vi "T90 main.vi"() -> ()   [LabVIEW 2020, in "T90.lvlib"]
uses:
  T90.lvlib
  Visualisierungs Elemente/Auswahlfeld.ctl
  Visualisierungs Elemente/Zahlen-Ausgabefeld.ctl
  Visualisierungs Elemente/Button.ctl
  Seiten/FT-IR/FGV FT-IR Gasliste Aktionen.ctl
  Aktion FGV T90.ctl
  Seiten/Gaszuordnung AO/FGV Gaszuordnung Grenzen&Einheit Aktion.ctl
  Aktion Zustandsautomat.ctl
  Messdaten/Aktionen FGV Messdaten.ctl
  Schedule Modul/Aktion FGV Testdaten sammeln.ctl
  Funktionstasten/Funktionstasten-Aktion.ctl
  Funktionstasten/Zustaende.ctl
  Funktionstasten/FGV Erweiterte Bedienung Aktion.ctl
  T90 konfig.vi
  Messdaten/Messdaten.lvlib
  Seiten/FT-IR/FT-IR.lvlib
  Allgemein/allgemeine Sub-VIs.lvlib
  Funktionstasten/Funktionstasten.lvlib
  Seiten/Gaszuordnung AO/Gaszuordnung AO.lvlib
  Sprachverwaltung/Sprachverwaltung.lvlib
  Linearisierung V2/Protokoll/Protokoll.lvlib
  Schedule Modul/Schedule Modul.lvlib
  cRIO/PC/Kommunikation mit cRIO.lvlib
panel:
  out "T90 PDF":waveform(sgl)(graph) caption="T90"
  out "Einheit 2":string caption="Einheit"
  out "Durchfluss FTIR":T1 format="%#.3g"
  out "Bestanden?":bool caption="Ergebnis 1"
  out "Ergebnis:":string
  out "T50:":T1 caption="T50 (Response Time):" format="%#.2g"
  out "Rise Time":T1 caption="T10 - T90 (Rise Time):" format="%#.1g"
  out "T90:":T1 caption="T90 (Response Time):" format="%#.1g"
  out "T10:":T1 caption="T10 (Delay Time):" format="%#.2g"
  out "Status":string
  out "Einheit":string
  out "aktuelle Wert":T1 caption="aktueller Wert" format="%#.3g"
  in  "Abbrechen":T2
  out "Gaskomponente":T3 caption="Komponente" items=["NO (350,3000) LP 191C", "NO2 (150) LP 191C (1of2)", "NO2 (2000) LP 191C (2of2)", "N2O (300) LP 191C (1of2)", "NH3 (300) LP 191C (1of2)", "NH3 (900,3000) LP 191C (2of2)", "HNCO (400) 191C", "H2O% (30) LP 191C", "Formaldehyde (70,500) LP 191C", "CO2 low% (4) LP 191C (2of2)", "CO2% (20) LP 191C (1of2)", "CO (700) LP 191C (1of3)", "CO% (1) LP 191C (2of3)", "Propylene (1000) LP 191C", "Aromatic HC C7 (500) LP 191C", "Ethylene (1000) LP 191C", "CH4 (250) LP 191C (1of2)", "CH4 (5000) LP 191C (2of2)", "Ethane (1000) LP 191C", "Acetylene (1000) LP 191C", "HNO2 (20) 191C", "MeOH (1000) 191C", "CO% (10) LP 191C (3of3)", "Formic Acid (100) 191C", "SO2 (500) LP 191C", "Acetaldehyde (1000) LP 191C", "COS (100) LP 191C", "1,3 butadiene (100) LP 191C", "Oil as Octane (200) LP 191C", "N2O (1000) LP 191C (2of2)", "Propane (200) LP 191C", "NO2 autorange (2000)", "CO autorange (100000)", "CH4 autorange (5000)", "NH3 autorange (3000)", "NOx autorange (3000)", "HCD (10000)", "NMHCD (10000)", "CO2% autorange (20)", "H2Oppm (300000)", "N2O autorange (1000)", "NMNEHCD (3000)", "Temp. Messzelle", "Druck Messzelle", "sBeam@2500", "Temp. HL zu FT-IR", "Temp. HL Extern SP1", "Austrittstemp. FT-IR", "Temp. Schaltschrank", "Konstant 0", "Konstant 50", "Konstant 100", "AK DUMMY"]
  out "T90":waveform(sgl)(graph)
  # "sec."
  # "sec."
  # "sec."
  # "sec."
  # "T90"
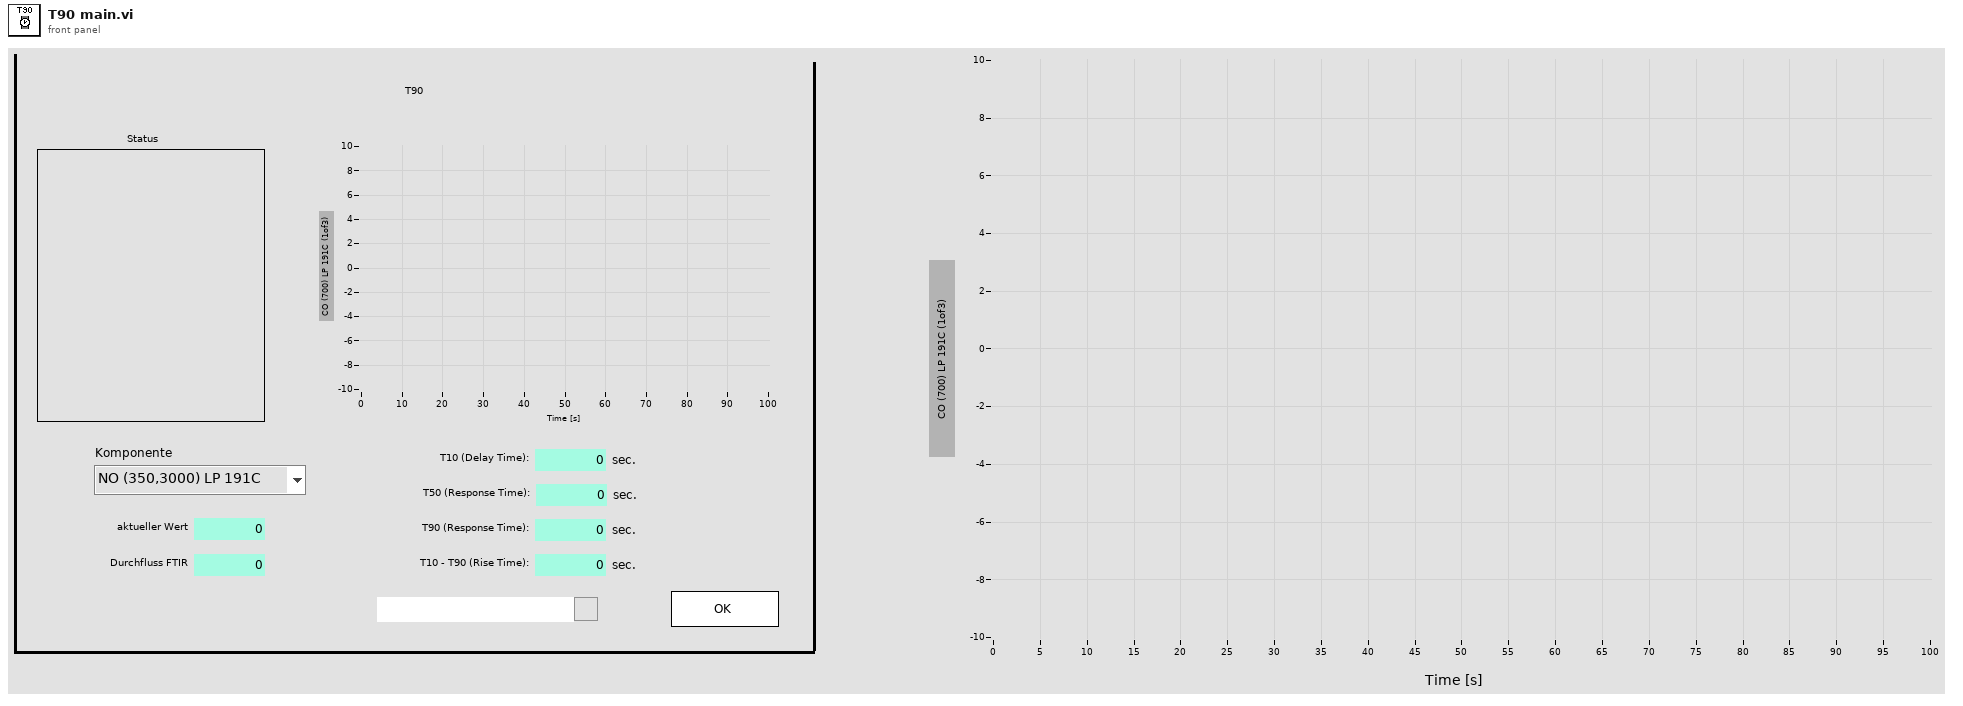
[diagram p1: front panel]
types:
  T1 = typedef "Zahlen-Ausgabefeld.ctl" = sgl
  T2 = typedef "Button.ctl" = bool
  T3 = typedef "Auswahlfeld.ctl" = u16
  T4 = typedef "Gaszuordnung AO.lvlib/FGV Gaszuordnung Grenzen&Einheit Aktion.ctl" = enum16{"Lesen", "Schreiben Min", "Schreiben Max", "Laden", "Speichern"}
  T5 = typedef "T90.lvlib/Aktion FGV T90.ctl" = enum16{"lesen", "schreiben", "laden", "speichern", "T90 aktiv", "T90 Entnahme aktiv", "Overflow Leak", "Pfad", "Zustand", "max. Responsetime"}
  T6 = typedef "FT-IR.lvlib/FGV FT-IR Gasliste Aktionen.ctl" = enum16{"lesen", "Gasliste FT-IR", "Gasliste ausgelesen", "laden", "speichern", "löschen"}
  T7 = typedef "T90.lvlib/Aktion Zustandsautomat.ctl" = enum16{"Initialisieren", "Warten", "Gas aufschalten", "Stabilisieren", "Volle Konzentration 1", "Berechnen", "Prüfung starten", "Prüfung", "Prüfung beenden", "keine Funktion"}
  T8 = typedef "T90.lvlib/T90 Gas Konfig.ctl" = cluster{"Gasflasche":T9, "Konfig Gasflasche":T10, "Auswahl":T3, "Sollwert":T11, "Abweichung":T11, "max. Responsetime":T11, "Modus:":T12, "Abschaltzeit":T11, "Stabilisierungszeit":T11, "Bearbeiter":string}
  T9 = typedef "System Einstellungen V2.lvlib/Gasflasche Auswahl.ctl" = u16
  T10 = typedef "System Einstellungen V2.lvlib/Konfig Gasflasche.ctl" = bool
  T11 = typedef "Zahlen-Eingabefeld.ctl" = sgl
  T12 = typedef "T90.lvlib/Zustand Auswahl.ctl" = u16
  T13 = typedef "String - Ausgabefeld.ctl" = string
  T14 = typedef "Messdaten.lvlib/Aktionen FGV Messdaten.ctl" = enum16{"lesen", "schreiben", "löschen", "Mittelwerte", "Komponente"}
  T15 = typedef "Schedule Modul.lvlib/Aktion FGV Testdaten sammeln.ctl" = enum16{"lesen", "Dichtheitstest", "CalGasTest", "T90", "Kalibrieren", "init", "Kalender Daten"}
  T16 = typedef "Verwaltung - cRIO.lvlib/Analog Eingaenge.ctl" = cluster{"AI0: Durchfluss FT-IR":sgl, "AI1: Druck Ausgang":sgl, "AI2: Umgebungsdruck":sgl, "AI3: Druck FT-IR":sgl, "AI4: Druck CalGas":sgl, "AI5: Reserve":sgl, "AI6: Reserve":sgl, "AI7: Reserve":sgl, "Rohwert Durchfluss FT-IR":sgl, "Rohwert Druck Ausgang":sgl, "Rohwert Umgebungsdruck":sgl, "Rohwert Druck FT-IR":sgl, "Rohwert Druck CalGas":sgl, "Rohwert AI5":sgl, "Rohwert AI6":sgl, "Rohwert AI7":sgl, "Rohwert Diffdruck mbar FTIR":sgl}
  T17 = cluster{"Signalverlauf":waveform(sgl), "T90":dbl, "T50":dbl, "T10":dbl, "Rise time ":dbl, "Bestanden?":bool}
  T18 = typedef "Schedule Modul.lvlib/Ergebnis T90.ctl" = cluster{"T90":waveform(sgl), "T10:":T1, "T50:":T1, "T90:":T1, "Rise Time":T1, "Leitungslänge":T11, "Fehler":bool}
  T19 = typedef "Funktionstasten.lvlib/FGV Erweiterte Bedienung Aktion.ctl" = enum16{"Lesen", "Initialisieren", "N2 zu PNS", "Chart wechsel"}
  T20 = typedef "Funktionstasten.lvlib/Zustaende.ctl" = enum16{"Standby", "Pause", "Eco", "Messen", "Kalibrieren", "Spülen Filter", "Spülen Leitung", "Umgebungsluft", "0-Gas", "Cal-Gas", "CG zu PNS", "-------------", "Init 1", "Init 2", "Init 3", "Init 4", "Messen vorbereiten", "Messen durchführen", "Exit"}
  T21 = typedef "Funktionstasten.lvlib/Funktionstasten-Aktion.ctl" = enum16{"Initialisieren", "Zustand setzen", "Taste gedrückt", "Fehler speichern", "Lesen", "Manuell", "Remote", "Bitparallel", "Samplepoint", "Zeit Prüfen", "reset Umschalten"}
  T22 = typedef "String - Eingabefeld.ctl" = string
  T23 = typedef "Pfad-Eingabefeld.ctl" = path
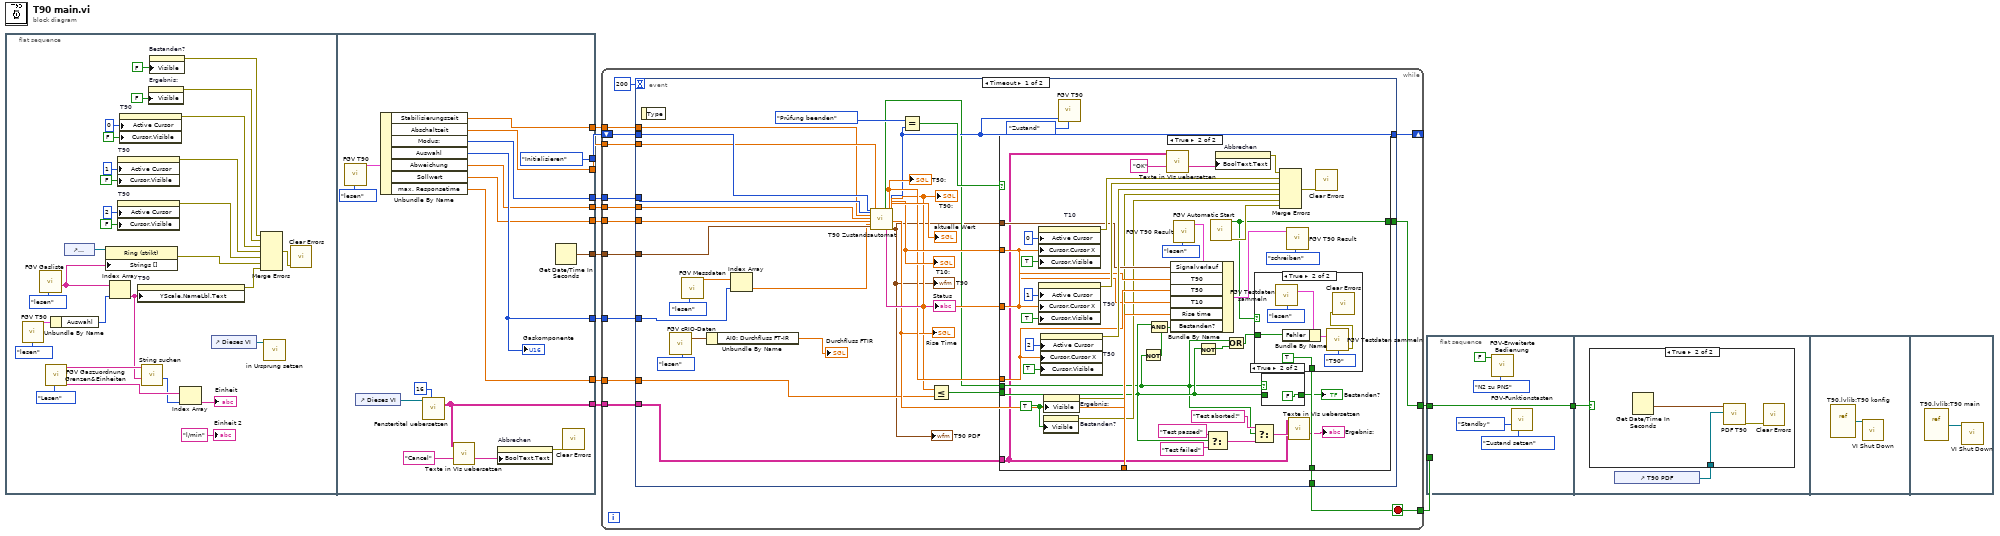
[diagram p0: block diagram]
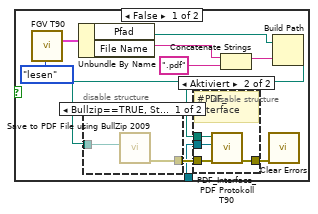
[diagram p2: hidden frame]
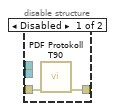
[diagram p3: hidden frame]
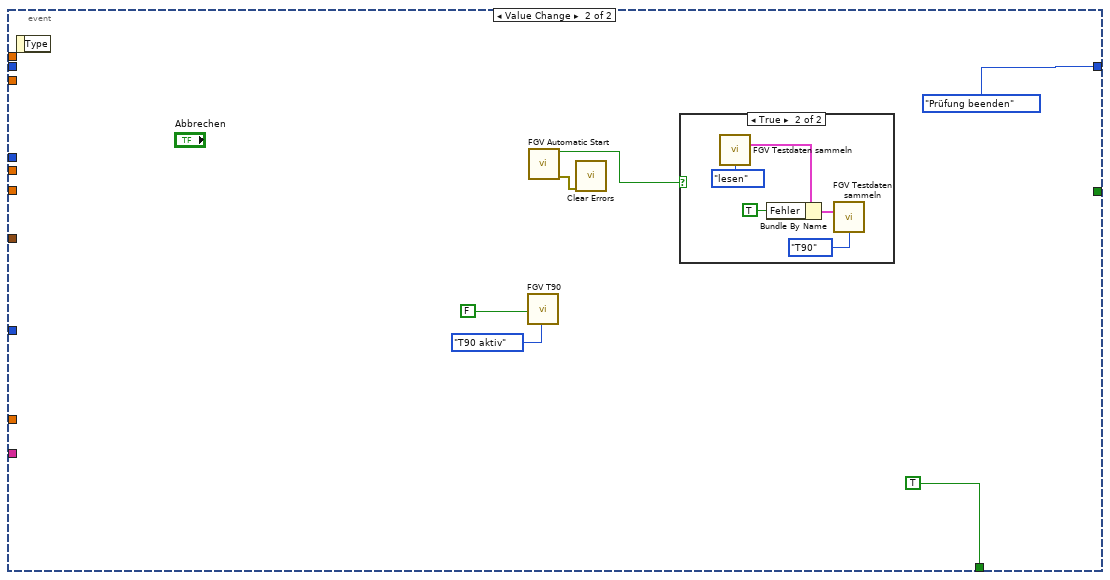
[diagram p8: hidden frame]
diagram:
  n1 = flat-sequence {
    tunnel: [w53] -> w13
    tunnel: [w51] -> w12
    tunnel: [w50] -> w11
    tunnel: [w59] -> w10
    tunnel: [w52] -> w9
    tunnel: [Aktion_Zustandsautomat."Initialisieren" ("Zustand")] -> w7
    tunnel: [w54] -> w6
    tunnel: [w49] -> w5
    tunnel: [w47] -> w4
    tunnel: [w44] -> w1
    frame #0 {
      n2 = call "FGV T90.vi"("Aktion"=Aktion_FGV_T90."lesen") -> ("Gas Konfig"=w16:T8)  [unwired: 20 in, 6 out]
      n3 = call "FGV Gasliste.vi"("Aktionen"=FGV_FT-IR_Gasliste_Aktionen."lesen") -> ("Aktuelle Gasliste gesamt"=w40:T13[])  [unwired: 8 in, 2 out]
      n4 = call "FGV Gaszuordnung Grenzen&Einheiten.vi"("Aktion"=FGV_Gaszuordnung_Grenzen&Einheit_Aktion."Lesen") -> ("Einheit neu"=w30:string[], "Namen neu"=w23:string[])  [unwired: 7 in, 2 out]
      n5 = Unbundle By Name(w16) -> ("Auswahl"=w15:T3)
      n6 = control-ref of="Gaskomponente"() -> (w42:refnum<vi>)
      n7 = property class="Ring (strikt)"(reference=w42, "Strings []"=w40) -> (error out=w38:errorcluster)  [unwired: 1 in, 1 out]
      n8 = Index Array(array=w40, index=w15) -> (element=w22:T13)
      n9 = property on="T90" class="SVGraph (strikt)"("Active Cursor"=u32 1 ("Aktiver Cursor"), "Cursor.Visible"=FALSE ("Cursor.Sichtbar")) -> (error out=w25:errorcluster)  [unwired: 2 in, 1 out]
      n10 = property on="T90" class="SVGraph (strikt)"("Active Cursor"=u32 2 ("Aktiver Cursor"), "Cursor.Visible"=FALSE ("Cursor.Sichtbar")) -> (error out=w26:errorcluster)  [unwired: 2 in, 1 out]
      n11 = property on="T90" class="SVGraph (strikt)"("Active Cursor"=u32 0 ("Aktiver Cursor"), "Cursor.Visible"=FALSE ("Cursor.Sichtbar")) -> (error out=w24:errorcluster)  [unwired: 2 in, 1 out]
      n12 = property on="T90" class="SVGraph (strikt)"("YScale.NameLbl.Text"=w22) -> (error out=w39:errorcluster)  [unwired: 2 in, 1 out]
      n13 = call "String suchen.vi"("Gasname"=w22, "Such-Namen"=w23) -> ("Index"=w21:i32)  [unwired: 8 in, 1 out]
      n14 = property on="Ergebnis:" class="Str"("Visible"=FALSE ("Sichtbar")) -> (error out=w20:errorcluster)  [unwired: 2 in, 1 out]
      n15 = property on="Bestanden?" class="Bool. (strikt)"("Visible"=FALSE ("Sichtbar")) -> (error out=w19:errorcluster)  [unwired: 2 in, 1 out]
      n16 = Index Array(array=w30, index=w21) -> (element=→"Einheit":string)
      n17 = control-ref of="Dieses VI"() -> (w32:refnum<vi>)
      n18 = Merge Errors(w19, w20, w24, w25, w26, w38, w39) -> (w37:errorcluster)
      n19 = call "in Ursprung setzen.vi"("VI Referenz"=w32) -> ()  [unwired: 10 in, 1 out]
      n20 = call <vilib>:"Clear Errors.vi"("error in (no error)"=w37) -> ()  [unwired: 5 in, 2 out]
      "Einheit 2" <- "l/min" ("Einheit 2")
    }
    frame #1 {
      n21 = call "FGV T90.vi"("Aktion"=Aktion_FGV_T90."lesen") -> ("Gas Konfig"=w55:T8)  [unwired: 20 in, 6 out]
      n22 = control-ref of="Dieses VI"() -> (w57:refnum<vi>)
      n23 = Unbundle By Name(w55) -> ("Stabilisierungszeit"=w44:T11, "Abschaltzeit"=w54:T11, "Modus:"=w53:T12, "Auswahl"=w52:T3, "Abweichung"=w51:T11, "Sollwert"=w50:T11, "max. Responsetime"=w49:T11)
      "Gaskomponente" <- w52
      n24 = call "Fenstertitel uebersetzen.vi"("Index (Seite)"=16, "Dieses VI"=w57) -> ("Sprachliste"=w47:string[][])  [unwired: 6 in, 3 out]
      n25 = call "Texte in VIs uebersetzen.vi"("Sprachliste"=w47, "String zum Übersetzen"="Cancel" ("Boolescher Text.Text")) -> ("String zum Übersetzen"=w45:string)  [unwired: 9 in, 4 out]
      n26 = property on="Abbrechen" class="Bool."("BoolText.Text"=w45) -> (error out=w46:errorcluster)  [unwired: 2 in, 1 out]
      n27 = Get Date/Time In Seconds() -> (seconds since 1Jan1904=w59:timestamp)
      n28 = call <vilib>:"Clear Errors.vi"("error in (no error)"=w46) -> ()  [unwired: 5 in, 2 out]
    }
  }
  n29 = while {
    shift-right: [w73] -> _
    shift-left: w7 -> [w72]
    tunnel: w13 -> [w71]
    tunnel: w12 -> [w70]
    tunnel: w11 -> [w69]
    tunnel: w10 -> [w68]
    tunnel: w9 -> [w67]
    tunnel: [w66] -> w8
    tunnel: w6 -> [w65]
    tunnel: w5 -> [w64]
    tunnel: w4 -> [w63]
    tunnel: [w62] -> w3
    tunnel: w1 -> [w61]
    stop <- w66 stop-if-true
    n30 = event shown="[0] Timeout" {
      selector: _ -> [_ _]
      dyn-events: _ -> [_ _]
      timeout: 200 -> [_ _]
      tunnel: [w85 TRUE] -> w66
      tunnel: [w82 Aktion_Zustandsautomat."Prüfung beenden" ("Zustand")] -> w73
      tunnel: w72 -> [w105 _]
      tunnel: w71 -> [w80 _]
      tunnel: w70 -> [w103 _]
      tunnel: w69 -> [w102 _]
      tunnel: w68 -> [w101 _]
      tunnel: w67 -> [w98 _]
      tunnel: w65 -> [w96 _]
      tunnel: w64 -> [w87 _]
      tunnel: w63 -> [w84 _]
      tunnel: [w83 _] -> w62
      tunnel: w61 -> [w79 _]
      event Timeout {
        n31 = event-data() -> ()  [unwired: 1 in, 1 out]
        n32 = call "FGV cRIO-Daten.vi"("Aktion"=enum16{"lesen", "schreiben"}."lesen") -> ("Analog Input"=w77:T16)  [unwired: 9 in, 9 out]
        n33 = call "FGV Messdaten.vi"("Aktionen"=Aktionen_FGV_Messdaten."lesen") -> ("Aktuelle Messwerte"=w99:sgl[])  [unwired: 6 in, 8 out]
        n34 = Unbundle By Name(w77) -> ("AI0: Durchfluss FT-IR"=→"Durchfluss FTIR":sgl)
        n35 = Index Array(array=w99, index=w98) -> (element=w97:sgl)
        n36 = call "T90 Zustandsautomat.vi"("Zustand"=w105, "Modus:"=w80, "Stabilisierungszeit"=w79, "Abweichung"=w103, "Sollwert"=w102, "IST-Wert"=w97, "Zeitstempel"=w101, "Abschaltzeit"=w96) -> ("Timeout?"=w81:bool, "Status"=→"Status":string, "T50"=w91:dbl, "Zustand"=w82:T7, "T90"=w88:dbl, "T10"=w92:dbl, "IST-Wert"=→"aktuelle Wert":T11, "Rise time"=w90:dbl, "Signalverlauf"=w75:waveform(sgl))  [unwired: 9 in, 2 out]
        "T90:" <- w88
        "T90" <- w75
        "T10:" <- w92
        "Rise Time" <- w90
        "T50:" <- w91
        "T90 PDF" <- w75
        n37 = Equal?(x=Aktion_Zustandsautomat."Prüfung beenden" ("Zustand"), y=w82) -> (x = y?=w93:bool)
        n38 = Less Or Equal?(x=w88, y=w87) -> (x <= y?=w86:bool)
        n39 = case shown="True" w93 {
          tunnel: w92 -> [_ w130]
          tunnel: w88 -> [_ w132]
          tunnel: w91 -> [_ w131]
          tunnel: w75 -> [_ w133]
          tunnel: w90 -> [_ w129]
          tunnel: w86 -> [_ w112]
          tunnel: [_ w122] -> w85
          tunnel: w84 -> [_ w106]
          tunnel: [_ w120] -> w83
          tunnel: w81 -> [_ w110]
          frame False {
          }
          frame True {
            w126 = TRUE ("Sichtbar")
            n40 = property on="T10" class="SVGraph (strikt)"("Active Cursor"=u32 0 ("Aktiver Cursor"), "Cursor.Cursor X"=w130, "Cursor.Visible"=TRUE ("Cursor.Sichtbar")) -> (error out=w143:errorcluster)  [unwired: 2 in, 1 out]
            n41 = property on="T90" class="SVGraph (strikt)"("Active Cursor"=u32 1 ("Aktiver Cursor"), "Cursor.Cursor X"=w132, "Cursor.Visible"=TRUE ("Cursor.Sichtbar")) -> (error out=w142:errorcluster)  [unwired: 2 in, 1 out]
            n42 = property on="T50" class="SVGraph (strikt)"("Active Cursor"=u32 2 ("Aktiver Cursor"), "Cursor.Cursor X"=w131, "Cursor.Visible"=TRUE ("Cursor.Sichtbar")) -> (error out=w138:errorcluster)  [unwired: 2 in, 1 out]
            n43 = property on="Bestanden?" class="Bool. (strikt)"("Visible"=w126) -> (error out=w124:errorcluster)  [unwired: 2 in, 1 out]
            n44 = property on="Ergebnis:" class="Str"("Visible"=w126) -> (error out=w125:errorcluster)  [unwired: 2 in, 1 out]
            n45 = Not(x=w110) -> (.not. x?=w111:bool)
            n46 = And(x=w112, y=w111) -> (x .and. y?=w113:bool)
            n47 = call "Texte in VIs uebersetzen.vi"("Sprachliste"=w106, "String zum Übersetzen"="OK" ("Boolescher Text.Text")) -> ("String zum Übersetzen"=w107:string)  [unwired: 9 in, 4 out]
            n48 = call "FGV T90 Result.vi"("Aktion"=enum16{"lesen", "schreiben"}."lesen") -> ("T90 Cluster out"=w135:T17)  [unwired: 10 in]
            n49 = Bundle By Name(cluster=w135, "Signalverlauf"=w133, "T90"=w132, "T50"=w131, "T10"=w130, "Rise time"=w129, "Bestanden?"=w113) -> (w134:T17)
            n50 = Not(x=w112) -> (.not. x?=w115:bool)
            n51 = Select(t="Test passed", s=w112, f="Test failed") -> (s? t:f=w118:string)
            n52 = call "FGV Automatic Start.vi"() -> ("Automaticstart"=w120:bool, "error out"=w123:errorcluster)  [unwired: 14 in]
            n53 = property on="Abbrechen" class="Bool."("BoolText.Text"=w107) -> (error out=w109:errorcluster)  [unwired: 2 in, 1 out]
            n54 = Or(x=w110, y=w115) -> (x .or. y?=w116:bool)
            n55 = Select(t="Test aborted!", s=w110, f=w118) -> (s? t:f=w117:string)
            n56 = case shown="True" w120 {
              tunnel: w116 -> [_ w150]
              tunnel: [_ TRUE] -> w122
              frame False {
              }
              frame True {
                n57 = call "FGV Testdaten sammeln.vi"("Aktion"=Aktion_FGV_Testdaten_sammeln."lesen") -> ("Ergebnis T90"=w156:T18)  [unwired: 9 in, 5 out]
                n58 = Bundle By Name(cluster=w156, "Fehler"=w150) -> (w155:T18)
                n59 = call "FGV Testdaten sammeln.vi"("Ergebnis T90"=w155, "Aktion"=Aktion_FGV_Testdaten_sammeln."T90") -> ("error out"=w152:errorcluster)  [unwired: 8 in, 5 out]
                n60 = call <vilib>:"Clear Errors.vi"("error in (no error)"=w152) -> ()  [unwired: 5 in, 2 out]
              }
            }
            n61 = case shown="True" w110 {
              tunnel: w112 -> [w148 _]
              tunnel: [w148 FALSE ("Timeout?")] -> w114
              frame False {
              }
              frame True {
              }
            }
            "Bestanden?" <- w114
            n62 = Merge Errors(w109, w143, w142, w138, w125, w124, w123) -> (w141:errorcluster)
            n63 = call "FGV T90 Result.vi"("Aktion"=enum16{"lesen", "schreiben"}."schreiben", "T90 Cluster in"=w134) -> ()  [unwired: 9 in, 1 out]
            n64 = call "Texte in VIs uebersetzen.vi"("Sprachliste"=w106, "String zum Übersetzen"=w117) -> ("String zum Übersetzen"=→"Ergebnis:":string)  [unwired: 9 in, 4 out]
            n65 = call <vilib>:"Clear Errors.vi"("error in (no error)"=w141) -> ()  [unwired: 5 in, 2 out]
          }
        }
        n66 = call "FGV T90.vi"("Zustand"=w82, "Aktion"=Aktion_FGV_T90."Zustand") -> ()  [unwired: 19 in, 7 out]
      }
      event Value Change {
        n67 = event-data() -> ()  [unwired: 1 in, 1 out]
        n68 = call "FGV T90.vi"("aktiv"=FALSE, "Aktion"=Aktion_FGV_T90."T90 aktiv") -> ()  [unwired: 19 in, 7 out]
        n69 = call "FGV Automatic Start.vi"() -> ("Automaticstart"=w158:bool, "error out"=w157:errorcluster)  [unwired: 14 in]
        n70 = call <vilib>:"Clear Errors.vi"("error in (no error)"=w157) -> ()  [unwired: 5 in, 2 out]
        n71 = case shown="True" w158 {
          frame False {
          }
          frame True {
            n72 = call "FGV Testdaten sammeln.vi"("Aktion"=Aktion_FGV_Testdaten_sammeln."lesen") -> ("Ergebnis T90"=w164:T18)  [unwired: 9 in, 5 out]
            n73 = Bundle By Name(cluster=w164, "Fehler"=TRUE) -> (w165:T18)
            n74 = call "FGV Testdaten sammeln.vi"("Ergebnis T90"=w165, "Aktion"=Aktion_FGV_Testdaten_sammeln."T90") -> ()  [unwired: 8 in, 6 out]
          }
        }
      }
    }
  }
  n75 = flat-sequence {
    tunnel: w8 -> [_]
    tunnel: w3 -> [w168]
    tunnel: [w168] -> w2
    tunnel: w2 -> [w174]
    frame #0 {
      n76 = call "FGV-Erweiterte Bedienung.vi"("Aktion"=FGV_Erweiterte_Bedienung_Aktion."N2 zu PNS", "N2 zu PNS"=FALSE) -> ()  [unwired: 8 in, 2 out]
      n77 = call "FGV-Funktionstasten.vi"("Zustand"=Zustaende."Standby", "Aktion"=Funktionstasten-Aktion."Zustand setzen") -> ()  [unwired: 6 in, 8 out]
    }
    frame #1 {
      n78 = control-ref of="T90 PDF"() -> (w173:refnum<vi>)
      n79 = case shown="True" w174 {
        tunnel: w173 -> [w175 w193]
        frame False {
          n80 = call "FGV T90.vi"("Aktion"=Aktion_FGV_T90."lesen") -> ("Protokolldaten"=w183:cluster{"File Name":T22, "Pfad":T23})  [unwired: 20 in, 6 out]
          n81 = Unbundle By Name(w183) -> ("Pfad"=w178:T23, "File Name"=w180:T22)
          n82 = Concatenate Strings(w180, ".pdf") -> (w181:string)
          n83 = Build Path(base path=w178, name or relative path=w181) -> (appended path=w176:path)
          n84 = disable-structure "Bedingte Deaktivierungsstruktur" shown="Bullzip==TRUE, Standard" {
            disable-tunnel: w176 -> [w192 _]
            disable-tunnel: [w191 _] -> w182
            frame condition #0 {
              n85 = call "Save to PDF File using BullZip 2009.vi"("Save PDF File Path"=w192) -> ("error out"=w191:errorcluster)  [unwired: 10 in]
            }
            frame condition #1 (active) {
            }
          }
          n86 = disable-structure shown="Aktiviert" {
            disable-tunnel: w182 -> [w186 w190]
            disable-tunnel: [w185 w189] -> w177
            disable-tunnel: w176 -> [_ w188]
            disable-tunnel: w175 -> [_ w187]
            frame Disabled {
              n87 = call "PDF Protokoll T90.vi"("error in (no error)"=w186) -> ("error out"=w185:errorcluster)  [unwired: 10 in]
            }
            frame Enabled {
              # "#PDF_Interface"
              n88 = call "PDF_Interface_PDF Protokoll T90.vi"("error in (no error)"=w190, "SVGraph Referenz"=w187, "Save PDF File Path"=w188) -> ("error out"=w189:errorcluster)  [unwired: 8 in]
            }
          }
          n89 = call <vilib>:"Clear Errors.vi"("error in (no error)"=w177) -> ()  [unwired: 5 in, 2 out]
        }
        frame True {
          n90 = Get Date/Time In Seconds() -> (seconds since 1Jan1904=w195:timestamp)
          n91 = call "PDF T90.vi"("SVGraph Referenz"=w193, "seconds since 1Jan1904"=w195) -> ("error out"=w194:errorcluster)  [unwired: 9 in]
          n92 = call <vilib>:"Clear Errors.vi"("error in (no error)"=w194) -> ()  [unwired: 5 in, 2 out]
        }
      }
    }
    frame #2 {
      n93 = vi-ref "T90.lvlib:T90 konfig.vi"() -> (w196:refnum<vi>)
      n94 = call "VI Shut Down.vi"("VI Referenz"=w196) -> ()  [unwired: 11 in]
    }
    frame #3 {
      n95 = vi-ref "T90.lvlib:T90 main.vi"() -> (w197:refnum<vi>)
      n96 = call "VI Shut Down.vi"("VI Referenz"=w197) -> ()  [unwired: 11 in]
    }
  }
